vi "Config Dev Span.vi"(8 "error in":errorcluster, 9 "Loss (0.2 jpF)":dbl=0.2 min=-1200.0 max=1200.0 format="%#_10f", 10 "Capacitance (2.0 pF)":dbl=2.0 min=-100000.0 max=100000.0 format="%#_10f", 11 "VISA resource name":refnum<visa-resource-name>) -> (0 "error out":errorcluster, 3 "VISA resource name out":refnum<visa-resource-name>)   [LabVIEW 2019, in "Andeen-Hagerling 2700(400 firmware).lvlib"]
doc: "Sets the span between the DBndLo and DBndUp in pF (or jpF)."
uses:
  Andeen-Hagerling 2700(400 firmware).lvlib
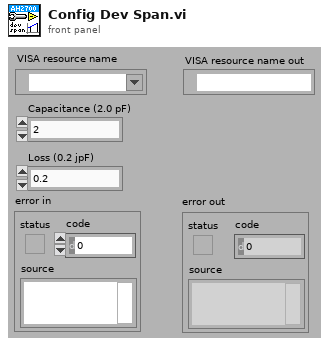
[diagram p1: front panel]
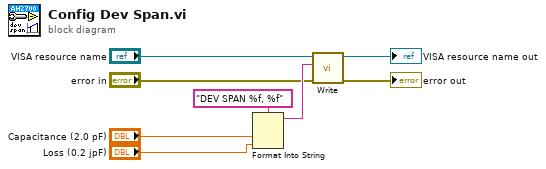
[diagram p0: block diagram]
diagram:
  n1 = Format Into String(format string="DEV SPAN %f, %f", "Capacitance (2.0 pF)", "Loss (0.2 jpF)") -> (resulting string=w7:string)  [unwired: 2 in, 1 out]
  n2 = call "Write.vi"("error in"="error in", "command"=w7, "VISA resource name"="VISA resource name") -> ("error out"=→"error out":errorcluster, "VISA resource name out"=→"VISA resource name out":refnum<visa-resource-name>)  [unwired: 7 in]
